vi "libssh2_sftp_last_error.vi"(8 "error in (no error)":errorcluster, 11 "sftp":T1) -> (0 "error out":errorcluster)   [LabVIEW 2013, in "libssh2.lvlib"]
doc: "Read the last SFTP-specific error.\n\nThis only works when libssh2 returned LIBSSH2_ERROR_SFTP_PROTOCOL in a previous call. Otherwise, the return value is undefined."
uses:
  libssh2.lvlib
  SFTP Refnum.ctl
  Global Settings.vi
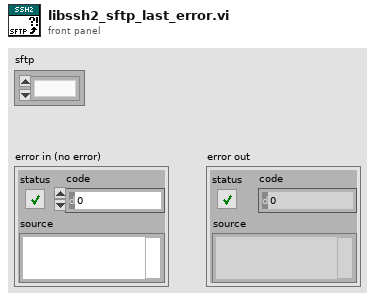
[diagram p1: front panel]
types:
  T1 = typedef "libssh2.lvlib/SFTP Refnum.ctl" = refnum<k1>
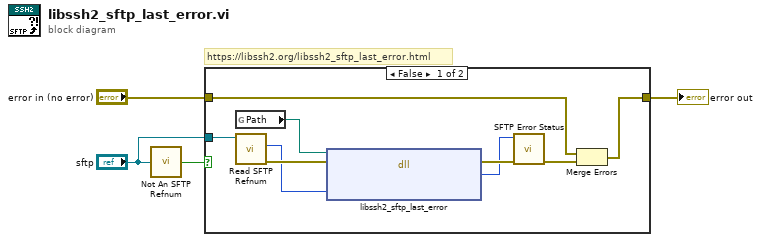
[diagram p0: block diagram]
diagram:
  # "https://libssh2.org/libssh2_sftp_last_error.html"
  n1 = call "Not An SFTP Refnum.vi"("sftp"="sftp") -> ("Not a SFTP Refnum?"=w4:bool)
  n2 = case shown="False" w4 {
    tunnel: "sftp" -> [w12 _]
    tunnel: [w5 w14] -> w3
    tunnel: "error in (no error)" -> [w7 w14]
    frame False {
      n3 = global read "Global Settings.vi" "Path"() -> (w13:path)
      n4 = call "Read SFTP Refnum.vi"("sftp"=w12) -> ("error out"=w11:errorcluster, "LIBSSH2_SFTP*"=w10:u64)  [unwired: 9 in]
      n5 = dll-call lib="?" fn="libssh2_sftp_last_error"(path in=w13, error in=w11, "sftp"=w10) -> (error out=w9:errorcluster, "return value"=w8:i32)  [unwired: 2 in, 1 out]
      n6 = call "SFTP Error Status.vi"("error in (no error)"=w9, "return value"=w8) -> ("error out"=w6:errorcluster)  [unwired: 8 in, 1 out]
      n7 = Merge Errors(w7, w6) -> (w5:errorcluster)
    }
    frame True {
    }
  }
  "error out" <- w3
